vi "GyroSampleSensorLoop.vi"   [LabVIEW 2018]
uses:
  GyroRxLoopData.ctl
  GyroRxLoopStates.ctl
  GyroSBITSample.ctl
  GyroLBITSample.ctl
  GyroSample.ctl
  GyroErrorSample.ctl
  GyroErrorCodes.ctl
  <vilib>/Platform/TimedLoop/XDataNode/timing_clust.ctl
  <vilib>/Platform/TimedLoop/XDataNode/nitl_modes.ctl
  <vilib>/Platform/TimedLoop/XDataNode/wakeup.ctl
  <vilib>/rvi/Emulation/niFpgaSctlEmulationGetInTimedLoop.vi
  <vilib>/rvi/Emulation/niFpgaEmulationReportErrorSimple.vi
  <vilib>/rvi/Emulation/niFpgaGetClockAttributes.vi
  <vilib>/rvi/Emulation/niFpgaCriticalErrorInLSC.vi
  <vilib>/rvi/Emulation/niFpgaEmulationIsFPGAContextNoSignature.vi
  <vilib>/rvi/errors/niFpgaSetErrorForExecOnDevCompSimple.vi
  <vilib>/rvi/eio/common/nirviEmuReportErrorAndStop.vi
  <vilib>/rvi/DataTransferAndStorage/Container/Common/niFpgaContainerGetUniqueNameForEmu.vi
  <vilib>/rvi/FIFO/Fifo_Resource/nirvififoEmulationSetSize.vi
  <vilib>/rvi/FIFO/Fifo_Resource/nirviFifoEmulationQueueMgr.vi
  <instcachedir>/0/nirviFifoEmulationQueueMgr_E5CAEC123FF24DC58D834DCA3CDAA9B5.lvgen/nirviFifoEmulationQueueMgr_E5CAEC123FF24DC58D834DCA3CDAA9B5_001.vi
  <vilib>/Utility/error.llb/Clear Errors.vi
  <vilib>/rvi/FIFO/Fifo_Resource/nirvififoEmulationCreateLock.vi
  <vilib>/rvi/Emulation/niFpgaProcessEmulError.vi
  <vilib>/rvi/FIFO/Fifo_Resource/nirvififoEmulationObtainLock.vi
  <vilib>/rvi/FIFO/Fifo_Resource/nirvififoEmulationReleaseLock.vi
  <vilib>/rvi/occurrence/nirviWaitOnOccurrenceBase.vi
  <vilib>/rvi/errors/nirviReportUnexpectedCaseInternalError.vi
  <vilib>/rvi/errors/nirviReportUnexpectedCaseInternalError (U32).vi
  <vilib>/rvi/eio/common/nirviEmuTemplateMethod_errors.vi
  <vilib>/rvi/Memory/Memory_Emulation/niFpgaMemoryEmulationCacheClearOnFirstRun.vi
  <vilib>/rvi/Memory/Memory_Emulation/nirvimemoryEmulationManagerCache_MakeExclusive.vi
  <vilib>/rvi/Memory/Memory_Emulation/niFpgaMemoryEmulationValidateCache.vi
  <vilib>/rvi/Memory/Memory_Emulation/nirvimemoryEmulationManagerCache_InsertValue.vi
  <vilib>/rvi/Memory/Memory_Emulation/nirvimemoryEmulationManagerCache_ReleaseExclusive.vi
  <vilib>/rvi/Memory/Memory_Emulation/nirvimemoryEmulationManagerCache_GetValue.vi
  <vilib>/rvi/Memory/Memory_Emulation/nirvimemoryEmulationManagerCache_SetValue.vi
  <vilib>/rvi/FIFO/Fifo_Resource/nirvififoEmulationDetermineInputValidOut.vi
  <instcachedir>/0/nirviFifoEmulationQueueMgr_E5CAEC123FF24DC58D834DCA3CDAA9B5.lvgen/nirviFifoEmulationQueueMgr_E5CAEC123FF24DC58D834DCA3CDAA9B5_009.vi
  <instcachedir>/0/nirviFifoEmulationQueueMgr_E5CAEC123FF24DC58D834DCA3CDAA9B5.lvgen/nirviFifoEmulationQueueMgr_E5CAEC123FF24DC58D834DCA3CDAA9B5_010.vi
  <instcachedir>/0/nirviFifoEmulationQueueMgr_E5CAEC123FF24DC58D834DCA3CDAA9B5.lvgen/nirviFifoEmulationQueueMgr_E5CAEC123FF24DC58D834DCA3CDAA9B5_002.vi
  <instcachedir>/0/nirviFifoEmulationQueueMgr_E5CAEC123FF24DC58D834DCA3CDAA9B5.lvgen/nirviFifoEmulationQueueMgr_E5CAEC123FF24DC58D834DCA3CDAA9B5_008.vi
  <instcachedir>/0/nirviFifoEmulationQueueMgr_E5CAEC123FF24DC58D834DCA3CDAA9B5.lvgen/nirviFifoEmulationQueueMgr_E5CAEC123FF24DC58D834DCA3CDAA9B5_011.vi
  <instcachedir>/0/nirviFifoEmulationQueueMgr_E5CAEC123FF24DC58D834DCA3CDAA9B5.lvgen/nirviFifoEmulationQueueMgr_E5CAEC123FF24DC58D834DCA3CDAA9B5_012.vi
  <vilib>/Platform/TimedLoop/XDataNode/XDataNode.xnode
  <vilib>/rvi/DataTransferAndStorage/Container/XNode/niFpgaContainer.xnode
  <vilib>/rvi/FIFO/Fifo_Resource/nirvififoEmulationRead.vi
  <vilib>/eio/EIONode/EIONode.xnode
  <vilib>/rvi/DataTransferAndStorage/Register/Emulation/niFpgaRegisterEmulation.vi
  <vilib>/rvi/FIFO/Fifo_Resource/nirvififoEmulationWrite.vi
  <vilib>/Platform/TimedLoop/XDataNode/XDNodeRunTimeDep.lvlib
types:
  T1 = typedef "GyroRxLoopData.ctl" = cluster{"State":T2, "Timestamp":u64, "Timeout":i32, "CRC":u32, "Checksum":u8, "IsLBIT":bool, "ReservedCount":u8, "SBITSample":T3, "LBITSample":T4, "Sample":T5, "ErrorSample":T6}
  T2 = typedef "GyroRxLoopStates.ctl" = enum16{"WaitForSilence", "ReadHeader3", "IgnoreASCIIResponse", "ReadNormalHeader2", "ReadNormalHeader1", "ReadBITHeader0", "ReadBIT0", "ReadBIT1", "ReadBIT2", "ReadBIT3", "ReadBIT4", "ReadBIT5", "ReadBIT6", "ReadBIT7", "ReadChecksum", "PrepareSBIT", "MoveSBIT", "PrepareLBIT", "MoveLBIT", "ReadSampleHeader0", "ReadSampleX3", "ReadSampleX2", "ReadSampleX1", "ReadSampleX0", "ReadSampleY3", "ReadSampleY2", "ReadSampleY1", "ReadSampleY0", "ReadSampleZ3", "ReadSampleZ2", "ReadSampleZ1", "ReadSampleZ0", "ReadSampleReserved", "ReadSampleStatus", "ReadSampleSequenceNumber", "ReadSampleTemperature1", "ReadSampleTemperature0", "ReadSampleCRC3", "ReadSampleCRC2", "ReadSampleCRC1", "ReadSampleCRC0", "VerifyCRC", "PrepareSample", "MoveSample", "ResponseHeaderError", "ResponseCRCError", "ResponseTimeoutError", "ResponseChecksumError", "PrepareErrorCode", "MoveErrorCode", "ClearCRC", "WaitForCRCCleared"}
  T3 = typedef "GyroSBITSample.ctl" = cluster{"Timestamp":u64, "TxBytes":u64, "RxBytes":u64, "TxFrames":u64, "RxFrames":u64, "BIT0":u8, "BIT1":u8, "BIT2":u8, "BIT3":u8, "BIT4":u8, "BIT5":u8}
  T4 = typedef "GyroLBITSample.ctl" = cluster{"Timestamp":u64, "TxBytes":u64, "RxBytes":u64, "TxFrames":u64, "RxFrames":u64, "BIT0":u8, "BIT1":u8, "BIT2":u8, "BIT3":u8, "BIT4":u8, "BIT5":u8, "BIT6":u8, "BIT7":u8}
  T5 = typedef "GyroSample.ctl" = cluster{"Timestamp":u64, "TxBytes":u64, "RxBytes":u64, "TxFrames":u64, "RxFrames":u64, "GyroX":u32, "GyroY":u32, "GyroZ":u32, "Status":u8, "SequenceNumber":u8, "Temperature":i16}
  T6 = typedef "GyroErrorSample.ctl" = cluster{"Timestamp":u64, "TxBytes":u64, "RxBytes":u64, "TxFrames":u64, "RxFrames":u64, "ErrorCode":T7}
  T7 = typedef "GyroErrorCodes.ctl" = enum8{"None", "ResponseHeaderError", "ResponseCRCError", "ResponseTimeoutError", "ResponseChecksumError"}
  T8 = typedef "XDNodeRunTimeDep.lvlib/timing_clust.ctl" = cluster{"Expected End [f-1]":u64, "Actual End [f-1]":u64, "Finished Late? [f-1]":bool, "Expected End [i-1]":u64, "Actual End [i-1]":u64, "Finished Late? [i-1]":bool, "Expected Start [i]":u64, "Actual Start [i]":u64, "Expected Start [f]":u64, "Actual Start [f]":u64, "Source Name":string, "Structure Name":string, "Period":i64, "Deadline":i64, "Offset":i64, "Start":i64, "Priority":i32, "Timeout":i32, "Mode":T9, "Wakeup Reason":T10, "Error":errorcluster, "Source Type":string, "Secondary Source Type":string, "Global End Time":u64, "Global Start Time":u64, "Frame Duration":u64, "Iteration Duration":u64, "Assigned CPU":i32, "I/O Scan Engine Mode":u32}
  T9 = typedef "XDNodeRunTimeDep.lvlib/nitl_modes.ctl" = enum32{"No Change", "Process missed periods, maintain original phase", "Discard missed periods, maintain original phase", "Process missed periods, ignore original phase", "Discard missed periods, ignore original phase"}
  T10 = typedef "XDNodeRunTimeDep.lvlib/wakeup.ctl" = enum32{"Normal", "Aborted", "Asynchronous wakeup", "Timing source error", "Timed loop error", "Timeout"}
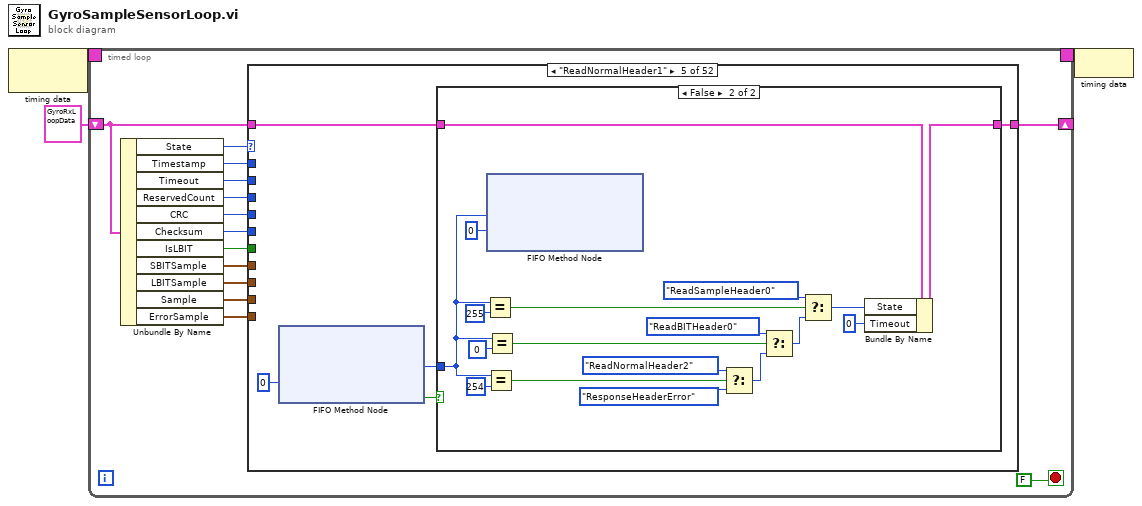
[diagram p0: block diagram]
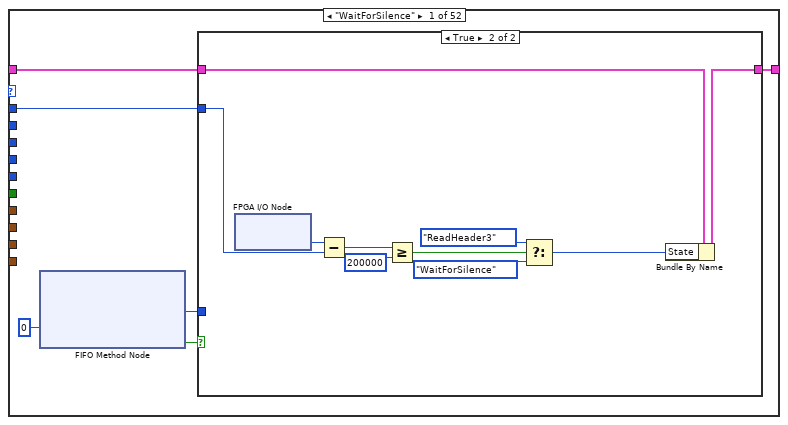
[diagram p2: hidden frame]
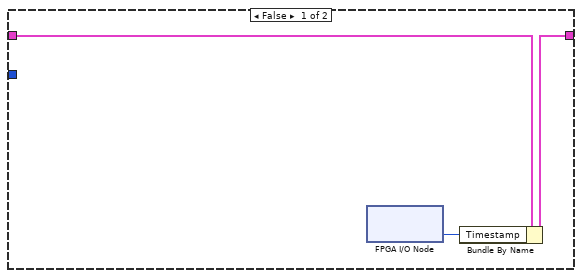
[diagram p3: hidden frame]
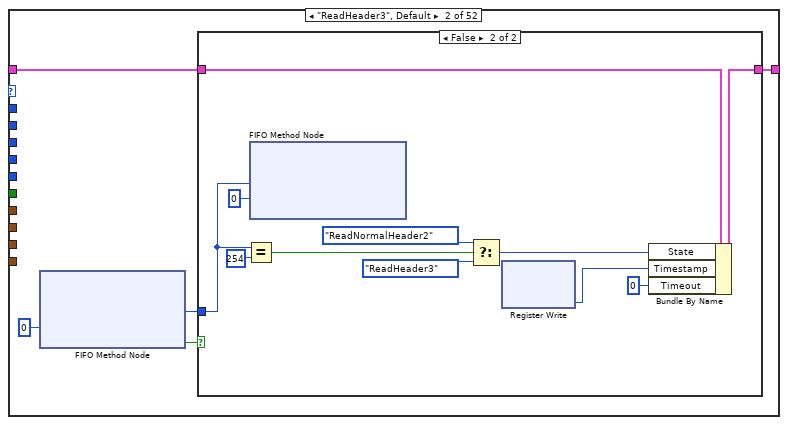
[diagram p4: hidden frame]
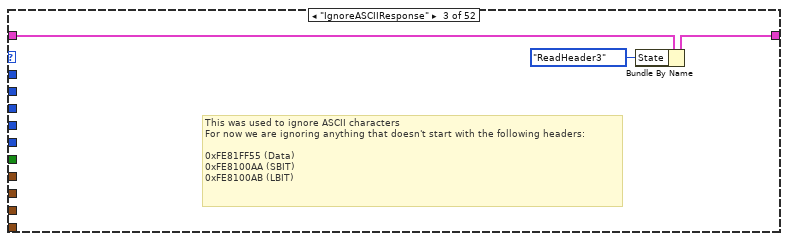
[diagram p6: hidden frame]
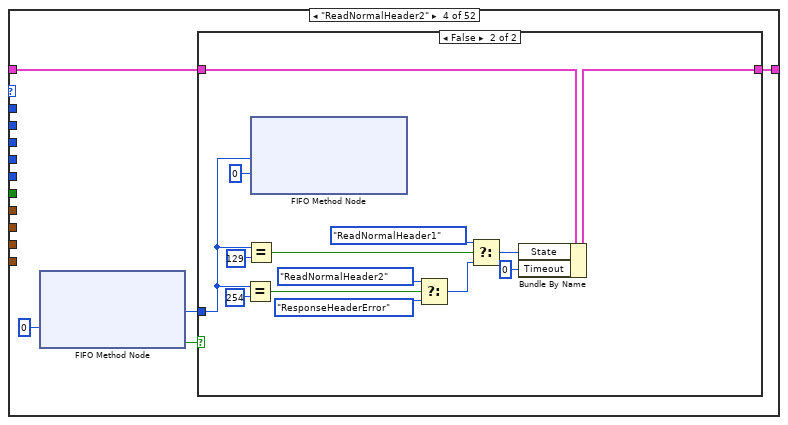
[diagram p7: hidden frame]
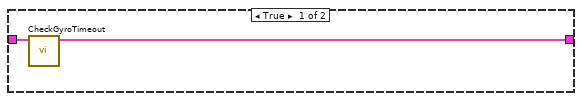
[diagram p8: hidden frame]
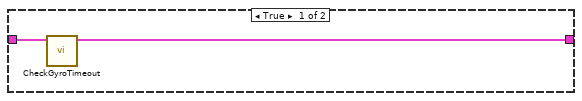
[diagram p9: hidden frame]
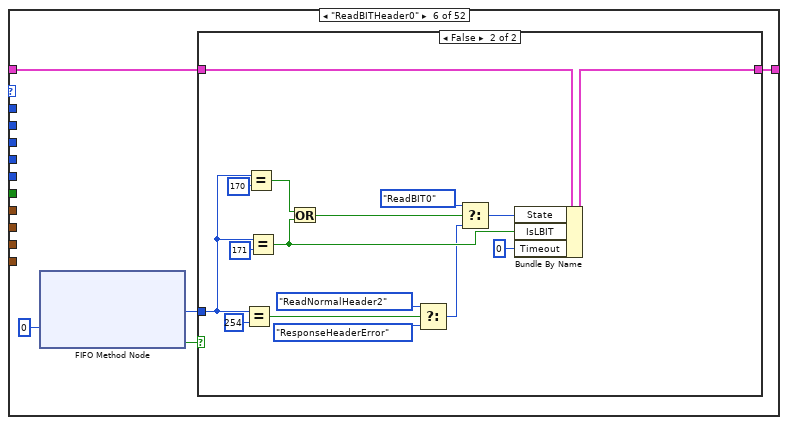
[diagram p10: hidden frame]
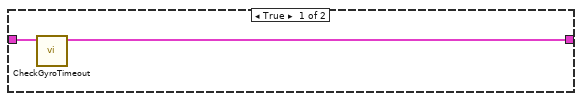
[diagram p11: hidden frame]
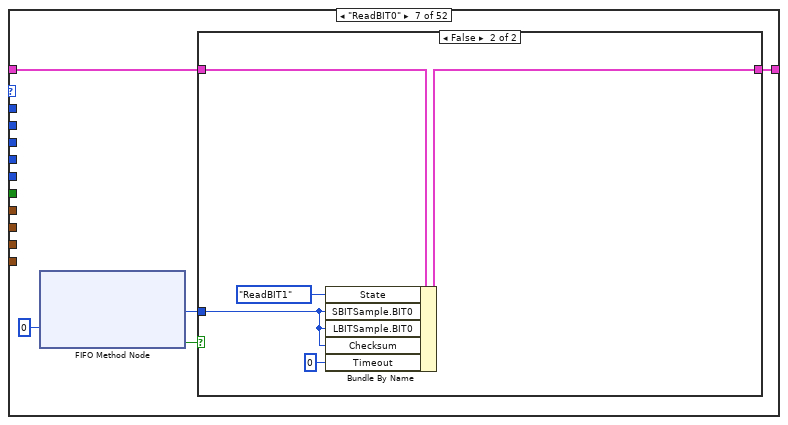
[diagram p12: hidden frame]
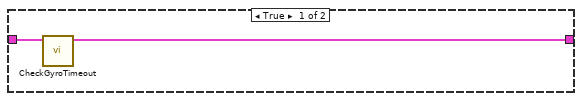
[diagram p13: hidden frame]
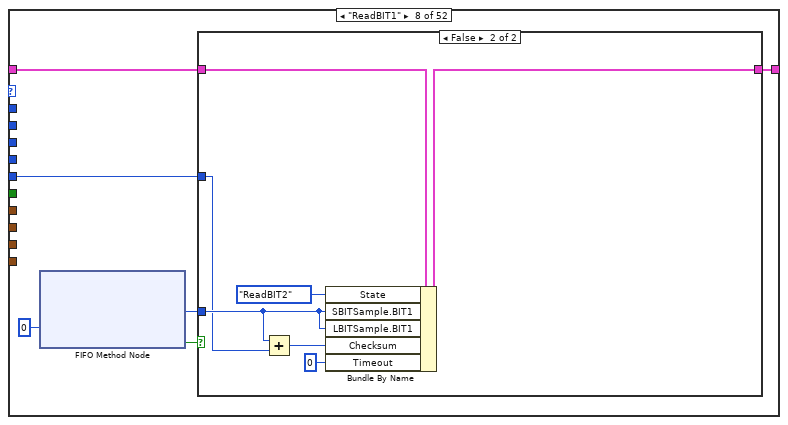
[diagram p14: hidden frame]
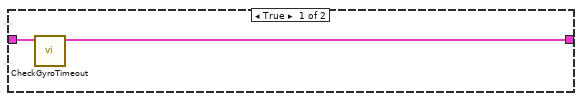
[diagram p15: hidden frame]
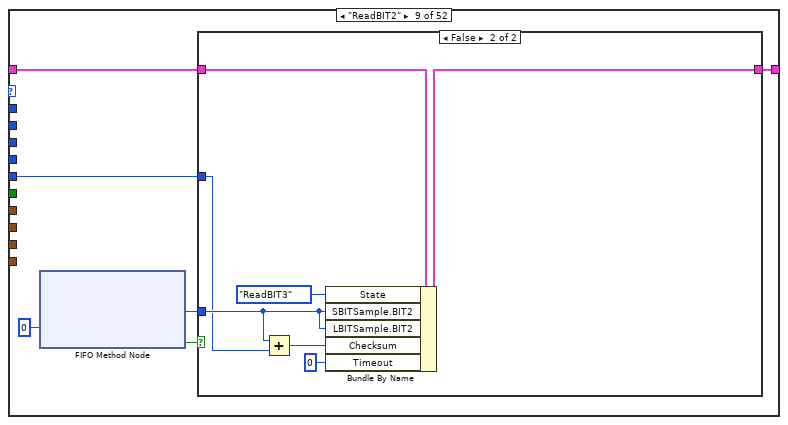
[diagram p16: hidden frame]
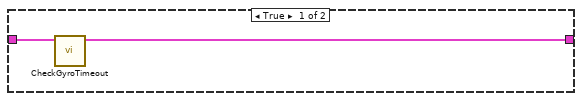
[diagram p17: hidden frame]
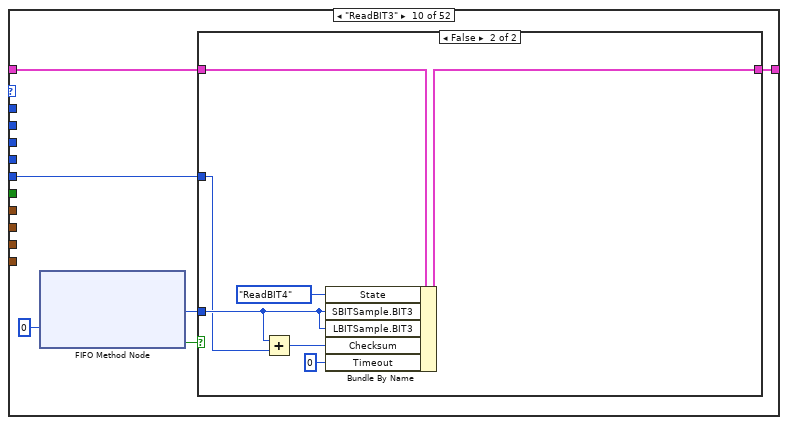
[diagram p18: hidden frame]
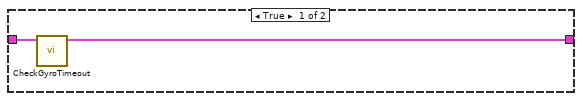
[diagram p19: hidden frame]
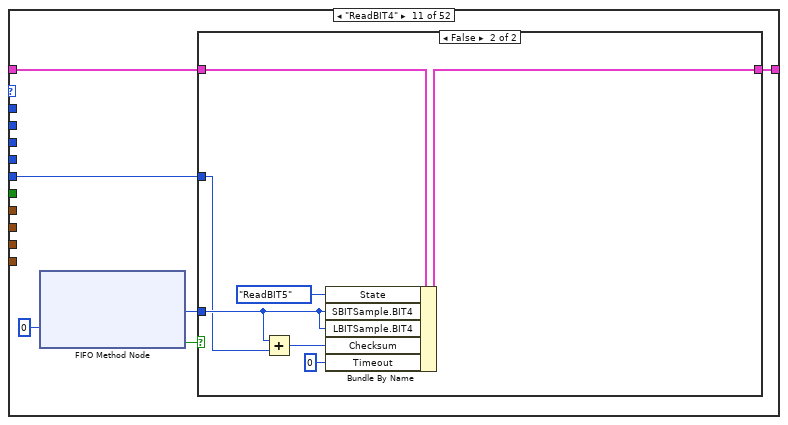
[diagram p20: hidden frame]
diagram:
  n1 = node-c288() -> (w3:T8)  [unwired: 1 in]
  n2 = timed-loop {
    timing: w3 -> [_]
    timing-out: [_] -> w2
    shift-right: [w17] -> _
    shift-left: T1 {"State"=enum."WaitForSilence", "Timestamp"=0, "Timeout"=0, "CRC"=0, "Checksum"=0, "IsLBIT"=FALSE, "ReservedCount"=0, "SBITSample"={"Timestamp"=0, "TxBytes"=0, "RxBytes"=0, "TxFrames"=0, "RxFrames"=0, "BIT0"=0, "BIT1"=0, "BIT2"=0, "BIT3"=0, "BIT4"=0, "BIT5"=0}, "LBITSample"={"Timestamp"=0, "TxBytes"=0, "RxBytes"=0, "TxFrames"=0, "RxFrames"=0, "BIT0"=0, "BIT1"=0, "BIT2"=0, "BIT3"=0, "BIT4"=0, "BIT5"=0, "BIT6"=0, "BIT7"=0}, "Sample"={"Timestamp"=0, "TxBytes"=0, "RxBytes"=0, "TxFrames"=0, "RxFrames"=0, "GyroX"=0, "GyroY"=0, "GyroZ"=0, "Status"=0, "SequenceNumber"=0, "Temperature"=0}, "ErrorSample"={"Timestamp"=0, "TxBytes"=0, "RxBytes"=0, "TxFrames"=0, "RxFrames"=0, "ErrorCode"=enum."None"}} ("GyroRxLoopData") -> [w16]
    stop <- FALSE stop-if-true
    n3 = Unbundle By Name(w16) -> ("State"=w15:T2, "Timestamp"=w14:u64, "Timeout"=w13:i32, "ReservedCount"=w9:u8, "CRC"=w12:u32, "Checksum"=w11:u8, "IsLBIT"=w10:bool, "SBITSample"=w8:T3, "LBITSample"=w7:T4, "Sample"=w6:T5, "ErrorSample"=w5:T6)
    n4 = case shown="\"ReadNormalHeader1\"" w15 {
      tunnel: [w19 w37 w55 w57 w78 w103 w126 w139 w154 w169 w184 w200 w218 w233 w249 w276 w281 w289 w294 w296 w317 w333 w351 w369 w385 w401 w419 w437 w453 w469 w487 w505 w523 w542 w555 w568 w584 w600 w618 w636 w654 w670 w692 w697 w701 w705 w709 w713 w721 w726 w731 w738] -> w17
      tunnel: w16 -> [w20 w38 w56 w58 w79 w104 w127 w140 w155 w170 w185 w201 w219 w234 w250 w277 w282 w290 w295 w297 w318 w334 w352 w370 w386 w402 w420 w438 w454 w470 w488 w506 w524 w543 w556 w569 w585 w601 w619 w637 w655 w671 w693 w698 w702 w706 w710 w714 w722 w727 w732 w739]
      tunnel: w14 -> [w18 _ _ _ _ _ _ _ _ _ _ _ _ _ _ w274 _ w287 _ _ _ _ _ _ _ _ _ _ _ _ _ _ _ _ _ _ _ _ _ _ _ _ w690 _ _ _ _ _ w719 _ _ _]
      tunnel: w13 -> [_ _ _ _ _ _ _ _ _ _ _ _ _ _ _ _ _ _ _ _ _ _ _ _ _ _ _ _ _ _ _ _ _ _ _ _ _ _ _ _ _ _ _ _ _ _ _ _ _ _ _ _]
      tunnel: w12 -> [_ _ _ _ _ _ _ _ _ _ _ _ _ _ _ _ _ _ _ _ _ _ _ _ _ _ _ _ _ _ _ _ _ _ _ _ _ _ w617 w635 w653 w669 _ _ _ _ _ _ _ _ _ _]
      tunnel: w11 -> [_ _ _ _ _ _ _ w138 w153 w168 w183 w199 w217 w232 w248 _ _ _ _ _ _ _ _ _ _ _ _ _ _ _ _ _ _ _ _ _ _ _ _ _ _ _ _ _ _ _ _ _ _ _ _ _]
      tunnel: w10 -> [_ _ _ _ _ _ _ _ _ _ _ w198 _ _ w247 _ _ _ _ _ _ _ _ _ _ _ _ _ _ _ _ _ _ _ _ _ _ _ _ _ _ _ _ _ _ _ _ _ _ _ _ _]
      tunnel: w9 -> [_ _ _ _ _ _ _ _ _ _ _ _ _ _ _ _ _ _ _ _ _ _ _ _ _ _ _ _ _ _ _ _ w522 _ _ _ _ _ _ _ _ _ _ _ _ _ _ _ _ _ _ _]
      tunnel: w8 -> [_ _ _ _ _ _ _ _ _ _ _ _ _ _ _ _ w278 _ _ _ _ _ _ _ _ _ _ _ _ _ _ _ _ _ _ _ _ _ _ _ _ _ _ _ _ _ _ _ _ _ _ _]
      tunnel: w7 -> [_ _ _ _ _ _ _ _ _ _ _ _ _ _ _ _ _ _ w291 _ _ _ _ _ _ _ _ _ _ _ _ _ _ _ _ _ _ _ _ _ _ _ _ _ _ _ _ _ _ _ _ _]
      tunnel: w6 -> [_ _ _ _ _ _ _ _ _ _ _ _ _ _ _ _ _ _ _ _ _ _ _ _ _ _ _ _ _ _ _ _ _ _ _ _ _ _ _ _ _ _ _ w695 _ _ _ _ _ _ _ _]
      tunnel: w5 -> [_ _ _ _ _ _ _ _ _ _ _ _ _ _ _ _ _ _ _ _ _ _ _ _ _ _ _ _ _ _ _ _ _ _ _ _ _ _ _ _ _ _ _ _ _ _ _ _ _ w724 _ _]
      frame "WaitForSilence" {
        n5 = xnode ("FIFO Method Node")("Timeout"=0) -> ("Element"=w22:u8, "Timed Out?"=w21:bool)  [unwired: 1 in, 1 out]
        n6 = case shown="True" w21 {
          tunnel: w22 -> [_ _]
          tunnel: w20 -> [w26 w36]
          tunnel: [w25 w35] -> w19
          tunnel: w18 -> [_ w33]
          frame False {
            n7 = xnode "FPGA I/O Node"() -> ("Time"=w24:u64)  [unwired: 1 in, 1 out]
            n8 = Bundle By Name(cluster=w26, "Timestamp"=w24) -> (w25:T1)
          }
          frame True {
            n9 = xnode "FPGA I/O Node"() -> ("Time"=w34:u64)  [unwired: 1 in, 1 out]
            n10 = Subtract(x=w34, y=w33) -> (x-y=w32:u64)
            n11 = Greater Or Equal?(x=w32, y=u64 200000) -> (x >= y?=w30:bool)
            n12 = Select(t=GyroRxLoopStates."ReadHeader3" ("State"), s=w30, f=GyroRxLoopStates."WaitForSilence" ("State")) -> (s? t:f=w27:T2)
            n13 = Bundle By Name(cluster=w36, "State"=w27) -> (w35:T1)
          }
        }
      }
      frame "ReadHeader3", Default {
        n14 = xnode ("FIFO Method Node")("Timeout"=0) -> ("Element"=w40:u8, "Timed Out?"=w39:bool)  [unwired: 1 in, 1 out]
        n15 = case shown="False" w39 {
          tunnel: w40 -> [_ w47]
          tunnel: w38 -> [w42 w50]
          tunnel: [w42 w49] -> w37
          frame True {
          }
          frame False {
            n16 = Equal?(x=w47, y=u8 254) -> (x = y?=w51:bool)
            n17 = xnode ("FIFO Method Node")("Element"=w47, "Timeout"=0) -> ()  [unwired: 1 in, 2 out]
            n18 = Select(t=GyroRxLoopStates."ReadNormalHeader2", s=w51, f=GyroRxLoopStates."ReadHeader3" ("t")) -> (s? t:f=w48:T2)
            n19 = xnode "Register Write"() -> ("Data"=w43:u64)  [unwired: 1 in, 1 out]
            n20 = Bundle By Name(cluster=w50, "State"=w48, "Timestamp"=w43, "Timeout"=0) -> (w49:T1)
          }
        }
      }
      frame "IgnoreASCIIResponse" {
        # "This was used to ignore ASCII characters\nFor now we are ignoring anything that doesn't start with the following headers:\n\n0xFE81FF55 (Data)\n0xFE8100AA (SBIT)\n0xFE8100AB (LBIT)"
        n21 = Bundle By Name(cluster=w56, "State"=GyroRxLoopStates."ReadHeader3") -> (w55:T1)
      }
      frame "ReadNormalHeader2" {
        n22 = xnode ("FIFO Method Node")("Timeout"=0) -> ("Element"=w60:u8, "Timed Out?"=w59:bool)  [unwired: 1 in, 1 out]
        n23 = case shown="False" w59 {
          tunnel: w60 -> [_ w69]
          tunnel: w58 -> [w63 w74]
          tunnel: [w62 w73] -> w57
          frame True {
            n24 = call "CheckGyroTimeout.vi"("GyroRxLoopData in"=w63) -> ("GyroRxLoopData out"=w62:T1)  [unwired: 10 in]
          }
          frame False {
            n25 = Equal?(x=w69, y=u8 254) -> (x = y?=w67:bool)
            n26 = Equal?(x=w69, y=u8 129) -> (x = y?=w75:bool)
            n27 = xnode ("FIFO Method Node")("Element"=w69, "Timeout"=0) -> ()  [unwired: 1 in, 2 out]
            n28 = Select(t=GyroRxLoopStates."ReadNormalHeader2", s=w67, f=GyroRxLoopStates."ResponseHeaderError") -> (s? t:f=w66:T2)
            n29 = Select(t=GyroRxLoopStates."ReadNormalHeader1", s=w75, f=w66) -> (s? t:f=w72:T2)
            n30 = Bundle By Name(cluster=w74, "State"=w72, "Timeout"=0) -> (w73:T1)
          }
        }
      }
      frame "ReadNormalHeader1" {
        n31 = xnode ("FIFO Method Node")("Timeout"=0) -> ("Element"=w81:u8, "Timed Out?"=w80:bool)  [unwired: 1 in, 1 out]
        n32 = case shown="False" w80 {
          tunnel: w81 -> [_ w87]
          tunnel: w79 -> [w84 w99]
          tunnel: [w83 w98] -> w78
          frame True {
            n33 = call "CheckGyroTimeout.vi"("GyroRxLoopData in"=w84) -> ("GyroRxLoopData out"=w83:T1)  [unwired: 10 in]
          }
          frame False {
            n34 = Equal?(x=w87, y=u8 255) -> (x = y?=w100:bool)
            n35 = Equal?(x=w87, y=u8 254) -> (x = y?=w90:bool)
            n36 = xnode ("FIFO Method Node")("Element"=w87, "Timeout"=0) -> ()  [unwired: 1 in, 2 out]
            n37 = Equal?(x=w87, y=u8 0) -> (x = y?=w95:bool)
            n38 = Select(t=GyroRxLoopStates."ReadNormalHeader2", s=w90, f=GyroRxLoopStates."ResponseHeaderError") -> (s? t:f=w86:T2)
            n39 = Select(t=GyroRxLoopStates."ReadBITHeader0" ("f"), s=w95, f=w86) -> (s? t:f=w93:T2)
            n40 = Select(t=GyroRxLoopStates."ReadSampleHeader0", s=w100, f=w93) -> (s? t:f=w97:T2)
            n41 = Bundle By Name(cluster=w99, "State"=w97, "Timeout"=0) -> (w98:T1)
          }
        }
      }
      frame "ReadBITHeader0" {
        n42 = xnode ("FIFO Method Node")("Timeout"=0) -> ("Element"=w106:u8, "Timed Out?"=w105:bool)  [unwired: 1 in, 1 out]
        n43 = case shown="False" w105 {
          tunnel: w106 -> [_ w113]
          tunnel: w104 -> [w109 w123]
          tunnel: [w108 w122] -> w103
          frame True {
            n44 = call "CheckGyroTimeout.vi"("GyroRxLoopData in"=w109) -> ("GyroRxLoopData out"=w108:T1)  [unwired: 10 in]
          }
          frame False {
            n45 = Equal?(x=w113, y=u8 254) -> (x = y?=w115:bool)
            n46 = Equal?(x=w113, y=u8 170) -> (x = y?=w119:bool)
            n47 = Equal?(x=w113, y=u8 171) -> (x = y?=w117:bool)
            n48 = Or(x=w119, y=w117) -> (x .or. y?=w118:bool)
            n49 = Select(t=GyroRxLoopStates."ReadNormalHeader2", s=w115, f=GyroRxLoopStates."ResponseHeaderError") -> (s? t:f=w111:T2)
            n50 = Select(t=GyroRxLoopStates."ReadBIT0", s=w118, f=w111) -> (s? t:f=w121:T2)
            n51 = Bundle By Name(cluster=w123, "State"=w121, "IsLBIT"=w117, "Timeout"=0) -> (w122:T1)
          }
        }
      }
      frame "ReadBIT0" {
        n52 = xnode ("FIFO Method Node")("Timeout"=0) -> ("Element"=w129:u8, "Timed Out?"=w128:bool)  [unwired: 1 in, 1 out]
        n53 = case shown="False" w128 {
          tunnel: w129 -> [_ w134]
          tunnel: w127 -> [w132 w137]
          tunnel: [w131 w136] -> w126
          frame True {
            n54 = call "CheckGyroTimeout.vi"("GyroRxLoopData in"=w132) -> ("GyroRxLoopData out"=w131:T1)  [unwired: 10 in]
          }
          frame False {
            n55 = Bundle By Name(cluster=w137, "State"=GyroRxLoopStates."ReadBIT1" ("t"), "SBITSample.BIT0"=w134, "LBITSample.BIT0"=w134, "Checksum"=w134, "Timeout"=0) -> (w136:T1)
          }
        }
      }
      frame "ReadBIT1" {
        n56 = xnode ("FIFO Method Node")("Timeout"=0) -> ("Element"=w142:u8, "Timed Out?"=w141:bool)  [unwired: 1 in, 1 out]
        n57 = case shown="False" w141 {
          tunnel: w142 -> [_ w149]
          tunnel: w140 -> [w145 w152]
          tunnel: [w144 w151] -> w139
          tunnel: w138 -> [_ w148]
          frame True {
            n58 = call "CheckGyroTimeout.vi"("GyroRxLoopData in"=w145) -> ("GyroRxLoopData out"=w144:T1)  [unwired: 10 in]
          }
          frame False {
            n59 = Add(x=w149, y=w148) -> (x+y=w147:u8)
            n60 = Bundle By Name(cluster=w152, "State"=GyroRxLoopStates."ReadBIT2" ("t"), "SBITSample.BIT1"=w149, "LBITSample.BIT1"=w149, "Checksum"=w147, "Timeout"=0) -> (w151:T1)
          }
        }
      }
      frame "ReadBIT2" {
        n61 = xnode ("FIFO Method Node")("Timeout"=0) -> ("Element"=w157:u8, "Timed Out?"=w156:bool)  [unwired: 1 in, 1 out]
        n62 = case shown="False" w156 {
          tunnel: w157 -> [_ w164]
          tunnel: w155 -> [w160 w167]
          tunnel: [w159 w166] -> w154
          tunnel: w153 -> [_ w163]
          frame True {
            n63 = call "CheckGyroTimeout.vi"("GyroRxLoopData in"=w160) -> ("GyroRxLoopData out"=w159:T1)  [unwired: 10 in]
          }
          frame False {
            n64 = Add(x=w164, y=w163) -> (x+y=w162:u8)
            n65 = Bundle By Name(cluster=w167, "State"=GyroRxLoopStates."ReadBIT3" ("t"), "SBITSample.BIT2"=w164, "LBITSample.BIT2"=w164, "Checksum"=w162, "Timeout"=0) -> (w166:T1)
          }
        }
      }
      frame "ReadBIT3" {
        n66 = xnode ("FIFO Method Node")("Timeout"=0) -> ("Element"=w172:u8, "Timed Out?"=w171:bool)  [unwired: 1 in, 1 out]
        n67 = case shown="False" w171 {
          tunnel: w172 -> [_ w179]
          tunnel: w170 -> [w175 w182]
          tunnel: [w174 w181] -> w169
          tunnel: w168 -> [_ w178]
          frame True {
            n68 = call "CheckGyroTimeout.vi"("GyroRxLoopData in"=w175) -> ("GyroRxLoopData out"=w174:T1)  [unwired: 10 in]
          }
          frame False {
            n69 = Add(x=w179, y=w178) -> (x+y=w177:u8)
            n70 = Bundle By Name(cluster=w182, "State"=GyroRxLoopStates."ReadBIT4" ("t"), "SBITSample.BIT3"=w179, "LBITSample.BIT3"=w179, "Checksum"=w177, "Timeout"=0) -> (w181:T1)
          }
        }
      }
      frame "ReadBIT4" {
        n71 = xnode ("FIFO Method Node")("Timeout"=0) -> ("Element"=w187:u8, "Timed Out?"=w186:bool)  [unwired: 1 in, 1 out]
        n72 = case shown="False" w186 {
          tunnel: w187 -> [_ w194]
          tunnel: w185 -> [w190 w197]
          tunnel: [w189 w196] -> w184
          tunnel: w183 -> [_ w193]
          frame True {
            n73 = call "CheckGyroTimeout.vi"("GyroRxLoopData in"=w190) -> ("GyroRxLoopData out"=w189:T1)  [unwired: 10 in]
          }
          frame False {
            n74 = Add(x=w194, y=w193) -> (x+y=w192:u8)
            n75 = Bundle By Name(cluster=w197, "State"=GyroRxLoopStates."ReadBIT5" ("t"), "SBITSample.BIT4"=w194, "LBITSample.BIT4"=w194, "Checksum"=w192, "Timeout"=0) -> (w196:T1)
          }
        }
      }
      frame "ReadBIT5" {
        n76 = xnode ("FIFO Method Node")("Timeout"=0) -> ("Element"=w203:u8, "Timed Out?"=w202:bool)  [unwired: 1 in, 1 out]
        n77 = case shown="False" w202 {
          tunnel: w203 -> [_ w214]
          tunnel: w201 -> [w206 w216]
          tunnel: [w205 w215] -> w200
          tunnel: w199 -> [_ w213]
          tunnel: w198 -> [_ w211]
          frame True {
            n78 = call "CheckGyroTimeout.vi"("GyroRxLoopData in"=w206) -> ("GyroRxLoopData out"=w205:T1)  [unwired: 10 in]
          }
          frame False {
            n79 = Add(x=w214, y=w213) -> (x+y=w212:u8)
            n80 = Select(t=GyroRxLoopStates."ReadBIT6", s=w211, f=GyroRxLoopStates."ReadChecksum") -> (s? t:f=w208:T2)
            n81 = Bundle By Name(cluster=w216, "State"=w208, "SBITSample.BIT5"=w214, "LBITSample.BIT5"=w214, "Checksum"=w212, "Timeout"=0) -> (w215:T1)
          }
        }
      }
      frame "ReadBIT6" {
        n82 = xnode ("FIFO Method Node")("Timeout"=0) -> ("Element"=w221:u8, "Timed Out?"=w220:bool)  [unwired: 1 in, 1 out]
        n83 = case shown="False" w220 {
          tunnel: w221 -> [_ w229]
          tunnel: w219 -> [w224 w231]
          tunnel: [w223 w230] -> w218
          tunnel: w217 -> [_ w228]
          frame True {
            n84 = call "CheckGyroTimeout.vi"("GyroRxLoopData in"=w224) -> ("GyroRxLoopData out"=w223:T1)  [unwired: 10 in]
          }
          frame False {
            n85 = Add(x=w229, y=w228) -> (x+y=w227:u8)
            n86 = Bundle By Name(cluster=w231, "State"=GyroRxLoopStates."ReadBIT7" ("t"), "LBITSample.BIT6"=w229, "Checksum"=w227, "Timeout"=0) -> (w230:T1)
          }
        }
      }
      frame "ReadBIT7" {
        n87 = xnode ("FIFO Method Node")("Timeout"=0) -> ("Element"=w236:u8, "Timed Out?"=w235:bool)  [unwired: 1 in, 1 out]
        n88 = case shown="False" w235 {
          tunnel: w236 -> [_ w244]
          tunnel: w234 -> [w239 w246]
          tunnel: [w238 w245] -> w233
          tunnel: w232 -> [_ w243]
          frame True {
            n89 = call "CheckGyroTimeout.vi"("GyroRxLoopData in"=w239) -> ("GyroRxLoopData out"=w238:T1)  [unwired: 10 in]
          }
          frame False {
            n90 = Add(x=w244, y=w243) -> (x+y=w242:u8)
            n91 = Bundle By Name(cluster=w246, "State"=GyroRxLoopStates."ReadChecksum" ("t"), "LBITSample.BIT7"=w244, "Checksum"=w242, "Timeout"=0) -> (w245:T1)
          }
        }
      }
      frame "ReadChecksum" {
        n92 = xnode ("FIFO Method Node")("Timeout"=0) -> ("Element"=w252:u8, "Timed Out?"=w251:bool)  [unwired: 1 in, 1 out]
        n93 = case shown="False" w251 {
          tunnel: w252 -> [_ w265]
          tunnel: w250 -> [w255 w267]
          tunnel: [w254 w266] -> w249
          tunnel: w248 -> [_ w264]
          tunnel: w247 -> [_ w263]
          frame True {
            n94 = call "CheckGyroTimeout.vi"("GyroRxLoopData in"=w255) -> ("GyroRxLoopData out"=w254:T1)  [unwired: 10 in]
          }
          frame False {
            n95 = Not Equal?(x=w264, y=w265) -> (x != y?=w257:bool)
            n96 = Select(t=GyroRxLoopStates."PrepareLBIT", s=w263, f=GyroRxLoopStates."PrepareSBIT" ("t")) -> (s? t:f=w259:T2)
            n97 = case shown="False" w257 {
              frame True {
              }
              frame False {
                n98 = xnode ("Register Read")() -> ("Data"=w269:u64)  [unwired: 1 in, 1 out]
                n99 = Increment(x=w269) -> (x+1=w268:u64)
                n100 = xnode ("Register Write")("Data"=w268) -> ()  [unwired: 1 in, 1 out]
              }
            }
            n101 = Select(t=GyroRxLoopStates."ResponseChecksumError", s=w257, f=w259) -> (s? t:f=w258:T2)
            n102 = Bundle By Name(cluster=w267, "State"=w258, "Timeout"=0) -> (w266:T1)
          }
        }
      }
      frame "PrepareSBIT" {
        n103 = xnode ("Register Read")() -> ("Data"=w273:u64)  [unwired: 1 in, 1 out]
        n104 = xnode ("Register Read")() -> ("Data"=w272:u64)  [unwired: 1 in, 1 out]
        n105 = xnode ("Register Read")() -> ("Data"=w271:u64)  [unwired: 1 in, 1 out]
        n106 = xnode ("Register Read")() -> ("Data"=w270:u64)  [unwired: 1 in, 1 out]
        n107 = Bundle By Name(cluster=w277, "State"=GyroRxLoopStates."MoveSBIT", "SBITSample.Timestamp"=w274, "SBITSample.TxBytes"=w273, "SBITSample.RxBytes"=w272, "SBITSample.TxFrames"=w271, "SBITSample.RxFrames"=w270) -> (w276:T1)
      }
      frame "MoveSBIT" {
        n108 = xnode ("FIFO Method Node")("Element"=w278, "Timeout"=0) -> ()  [unwired: 1 in, 2 out]
        n109 = Bundle By Name(cluster=w282, "State"=GyroRxLoopStates."ClearCRC") -> (w281:T1)
      }
      frame "PrepareLBIT" {
        n110 = xnode ("Register Read")() -> ("Data"=w286:u64)  [unwired: 1 in, 1 out]
        n111 = xnode ("Register Read")() -> ("Data"=w285:u64)  [unwired: 1 in, 1 out]
        n112 = xnode ("Register Read")() -> ("Data"=w284:u64)  [unwired: 1 in, 1 out]
        n113 = xnode ("Register Read")() -> ("Data"=w283:u64)  [unwired: 1 in, 1 out]
        n114 = Bundle By Name(cluster=w290, "State"=GyroRxLoopStates."MoveLBIT", "LBITSample.Timestamp"=w287, "LBITSample.TxBytes"=w286, "LBITSample.RxBytes"=w285, "LBITSample.TxFrames"=w284, "LBITSample.RxFrames"=w283) -> (w289:T1)
      }
      frame "MoveLBIT" {
        n115 = xnode ("FIFO Method Node")("Element"=w291, "Timeout"=0) -> ()  [unwired: 1 in, 2 out]
        n116 = Bundle By Name(cluster=w295, "State"=GyroRxLoopStates."ClearCRC") -> (w294:T1)
      }
      frame "ReadSampleHeader0" {
        n117 = xnode ("FIFO Method Node")("Timeout"=0) -> ("Element"=w299:u8, "Timed Out?"=w298:bool)  [unwired: 1 in, 1 out]
        n118 = case shown="False" w298 {
          tunnel: w299 -> [_ w305]
          tunnel: w297 -> [w302 w314]
          tunnel: [w301 w313] -> w296
          frame True {
            n119 = call "CheckGyroTimeout.vi"("GyroRxLoopData in"=w302) -> ("GyroRxLoopData out"=w301:T1)  [unwired: 10 in]
          }
          frame False {
            n120 = xnode ("FIFO Method Node")("Element"=w305, "Timeout"=0) -> ()  [unwired: 1 in, 2 out]
            n121 = Equal?(x=w305, y=u8 85) -> (x = y?=w311:bool)
            n122 = Equal?(x=w305, y=u8 254) -> (x = y?=w308:bool)
            n123 = Select(t=GyroRxLoopStates."ReadNormalHeader2", s=w308, f=GyroRxLoopStates."ResponseHeaderError") -> (s? t:f=w304:T2)
            n124 = Select(t=GyroRxLoopStates."ReadSampleX3", s=w311, f=w304) -> (s? t:f=w312:T2)
            n125 = Bundle By Name(cluster=w314, "State"=w312, "Timeout"=0) -> (w313:T1)
          }
        }
      }
      frame "ReadSampleX3" {
        n126 = xnode ("FIFO Method Node")("Timeout"=0) -> ("Element"=w320:u8, "Timed Out?"=w319:bool)  [unwired: 1 in, 1 out]
        n127 = case shown="False" w319 {
          tunnel: w320 -> [_ w329]
          tunnel: w318 -> [w323 w326]
          tunnel: [w322 w332] -> w317
          frame True {
            n128 = call "CheckGyroTimeout.vi"("GyroRxLoopData in"=w323) -> ("GyroRxLoopData out"=w322:T1)  [unwired: 10 in]
          }
          frame False {
            n129 = To Unsigned Long Integer(number=w329) -> (unsigned 32bit integer=w328:u32)
            n130 = xnode ("FIFO Method Node")("Element"=w329, "Timeout"=0) -> ()  [unwired: 1 in, 2 out]
            n131 = Logical Shift(y=i16 24, x=w328) -> (x << y=w325:u32)
            n132 = Bundle By Name(cluster=w326, "State"=GyroRxLoopStates."ReadSampleX2" ("t"), "Sample.GyroX"=w325, "Timeout"=0) -> (w332:T1)
          }
        }
      }
      frame "ReadSampleX2" {
        n133 = xnode ("FIFO Method Node")("Timeout"=0) -> ("Element"=w336:u8, "Timed Out?"=w335:bool)  [unwired: 1 in, 1 out]
        n134 = case shown="False" w335 {
          tunnel: w336 -> [_ w347]
          tunnel: w334 -> [w339 w344]
          tunnel: [w338 w350] -> w333
          frame True {
            n135 = call "CheckGyroTimeout.vi"("GyroRxLoopData in"=w339) -> ("GyroRxLoopData out"=w338:T1)  [unwired: 10 in]
          }
          frame False {
            n136 = Unbundle By Name(w344) -> ("Sample.GyroX"=w343:u32)
            n137 = To Unsigned Long Integer(number=w347) -> (unsigned 32bit integer=w346:u32)
            n138 = xnode ("FIFO Method Node")("Element"=w347, "Timeout"=0) -> ()  [unwired: 1 in, 2 out]
            n139 = Logical Shift(y=i16 16, x=w346) -> (x << y=w342:u32)
            n140 = Or(x=w343, y=w342) -> (x .or. y?=w341:u32)
            n141 = Bundle By Name(cluster=w344, "State"=GyroRxLoopStates."ReadSampleX1" ("t"), "Sample.GyroX"=w341, "Timeout"=0) -> (w350:T1)
          }
        }
      }
      frame "ReadSampleX1" {
        n142 = xnode ("FIFO Method Node")("Timeout"=0) -> ("Element"=w354:u8, "Timed Out?"=w353:bool)  [unwired: 1 in, 1 out]
        n143 = case shown="False" w353 {
          tunnel: w354 -> [_ w365]
          tunnel: w352 -> [w357 w362]
          tunnel: [w356 w368] -> w351
          frame True {
            n144 = call "CheckGyroTimeout.vi"("GyroRxLoopData in"=w357) -> ("GyroRxLoopData out"=w356:T1)  [unwired: 10 in]
          }
          frame False {
            n145 = Unbundle By Name(w362) -> ("Sample.GyroX"=w361:u32)
            n146 = To Unsigned Long Integer(number=w365) -> (unsigned 32bit integer=w364:u32)
            n147 = xnode ("FIFO Method Node")("Element"=w365, "Timeout"=0) -> ()  [unwired: 1 in, 2 out]
            n148 = Logical Shift(y=i16 8, x=w364) -> (x << y=w360:u32)
            n149 = Or(x=w361, y=w360) -> (x .or. y?=w359:u32)
            n150 = Bundle By Name(cluster=w362, "State"=GyroRxLoopStates."ReadSampleX0" ("t"), "Sample.GyroX"=w359, "Timeout"=0) -> (w368:T1)
          }
        }
      }
      frame "ReadSampleX0" {
        n151 = xnode ("FIFO Method Node")("Timeout"=0) -> ("Element"=w372:u8, "Timed Out?"=w371:bool)  [unwired: 1 in, 1 out]
        n152 = case shown="False" w371 {
          tunnel: w372 -> [_ w381]
          tunnel: w370 -> [w375 w380]
          tunnel: [w374 w384] -> w369
          frame True {
            n153 = call "CheckGyroTimeout.vi"("GyroRxLoopData in"=w375) -> ("GyroRxLoopData out"=w374:T1)  [unwired: 10 in]
          }
          frame False {
            n154 = Unbundle By Name(w380) -> ("Sample.GyroX"=w379:u32)
            n155 = To Unsigned Long Integer(number=w381) -> (unsigned 32bit integer=w378:u32)
            n156 = xnode ("FIFO Method Node")("Element"=w381, "Timeout"=0) -> ()  [unwired: 1 in, 2 out]
            n157 = Or(x=w379, y=w378) -> (x .or. y?=w377:u32)
            n158 = Bundle By Name(cluster=w380, "State"=GyroRxLoopStates."ReadSampleY3" ("t"), "Sample.GyroX"=w377, "Timeout"=0) -> (w384:T1)
          }
        }
      }
      frame "ReadSampleY3" {
        n159 = xnode ("FIFO Method Node")("Timeout"=0) -> ("Element"=w388:u8, "Timed Out?"=w387:bool)  [unwired: 1 in, 1 out]
        n160 = case shown="False" w387 {
          tunnel: w388 -> [_ w397]
          tunnel: w386 -> [w391 w394]
          tunnel: [w390 w400] -> w385
          frame True {
            n161 = call "CheckGyroTimeout.vi"("GyroRxLoopData in"=w391) -> ("GyroRxLoopData out"=w390:T1)  [unwired: 10 in]
          }
          frame False {
            n162 = To Unsigned Long Integer(number=w397) -> (unsigned 32bit integer=w396:u32)
            n163 = xnode ("FIFO Method Node")("Element"=w397, "Timeout"=0) -> ()  [unwired: 1 in, 2 out]
            n164 = Logical Shift(y=i16 24, x=w396) -> (x << y=w393:u32)
            n165 = Bundle By Name(cluster=w394, "State"=GyroRxLoopStates."ReadSampleY2" ("t"), "Sample.GyroY"=w393, "Timeout"=0) -> (w400:T1)
          }
        }
      }
      frame "ReadSampleY2" {
        n166 = xnode ("FIFO Method Node")("Timeout"=0) -> ("Element"=w404:u8, "Timed Out?"=w403:bool)  [unwired: 1 in, 1 out]
        n167 = case shown="False" w403 {
          tunnel: w404 -> [_ w415]
          tunnel: w402 -> [w407 w412]
          tunnel: [w406 w418] -> w401
          frame True {
            n168 = call "CheckGyroTimeout.vi"("GyroRxLoopData in"=w407) -> ("GyroRxLoopData out"=w406:T1)  [unwired: 10 in]
          }
          frame False {
            n169 = Unbundle By Name(w412) -> ("Sample.GyroY"=w411:u32)
            n170 = To Unsigned Long Integer(number=w415) -> (unsigned 32bit integer=w414:u32)
            n171 = xnode ("FIFO Method Node")("Element"=w415, "Timeout"=0) -> ()  [unwired: 1 in, 2 out]
            n172 = Logical Shift(y=i16 16, x=w414) -> (x << y=w410:u32)
            n173 = Or(x=w411, y=w410) -> (x .or. y?=w409:u32)
            n174 = Bundle By Name(cluster=w412, "State"=GyroRxLoopStates."ReadSampleY1" ("t"), "Sample.GyroY"=w409, "Timeout"=0) -> (w418:T1)
          }
        }
      }
      frame "ReadSampleY1" {
        n175 = xnode ("FIFO Method Node")("Timeout"=0) -> ("Element"=w422:u8, "Timed Out?"=w421:bool)  [unwired: 1 in, 1 out]
        n176 = case shown="False" w421 {
          tunnel: w422 -> [_ w433]
          tunnel: w420 -> [w425 w430]
          tunnel: [w424 w436] -> w419
          frame True {
            n177 = call "CheckGyroTimeout.vi"("GyroRxLoopData in"=w425) -> ("GyroRxLoopData out"=w424:T1)  [unwired: 10 in]
          }
          frame False {
            n178 = Unbundle By Name(w430) -> ("Sample.GyroY"=w429:u32)
            n179 = To Unsigned Long Integer(number=w433) -> (unsigned 32bit integer=w432:u32)
            n180 = xnode ("FIFO Method Node")("Element"=w433, "Timeout"=0) -> ()  [unwired: 1 in, 2 out]
            n181 = Logical Shift(y=i16 8, x=w432) -> (x << y=w428:u32)
            n182 = Or(x=w429, y=w428) -> (x .or. y?=w427:u32)
            n183 = Bundle By Name(cluster=w430, "State"=GyroRxLoopStates."ReadSampleY0" ("t"), "Sample.GyroY"=w427, "Timeout"=0) -> (w436:T1)
          }
        }
      }
      frame "ReadSampleY0" {
        n184 = xnode ("FIFO Method Node")("Timeout"=0) -> ("Element"=w440:u8, "Timed Out?"=w439:bool)  [unwired: 1 in, 1 out]
        n185 = case shown="False" w439 {
          tunnel: w440 -> [_ w449]
          tunnel: w438 -> [w443 w448]
          tunnel: [w442 w452] -> w437
          frame True {
            n186 = call "CheckGyroTimeout.vi"("GyroRxLoopData in"=w443) -> ("GyroRxLoopData out"=w442:T1)  [unwired: 10 in]
          }
          frame False {
            n187 = Unbundle By Name(w448) -> ("Sample.GyroY"=w447:u32)
            n188 = To Unsigned Long Integer(number=w449) -> (unsigned 32bit integer=w446:u32)
            n189 = xnode ("FIFO Method Node")("Element"=w449, "Timeout"=0) -> ()  [unwired: 1 in, 2 out]
            n190 = Or(x=w447, y=w446) -> (x .or. y?=w445:u32)
            n191 = Bundle By Name(cluster=w448, "State"=GyroRxLoopStates."ReadSampleZ3" ("t"), "Sample.GyroY"=w445, "Timeout"=0) -> (w452:T1)
          }
        }
      }
      frame "ReadSampleZ3" {
        n192 = xnode ("FIFO Method Node")("Timeout"=0) -> ("Element"=w456:u8, "Timed Out?"=w455:bool)  [unwired: 1 in, 1 out]
        n193 = case shown="False" w455 {
          tunnel: w456 -> [_ w465]
          tunnel: w454 -> [w459 w462]
          tunnel: [w458 w468] -> w453
          frame True {
            n194 = call "CheckGyroTimeout.vi"("GyroRxLoopData in"=w459) -> ("GyroRxLoopData out"=w458:T1)  [unwired: 10 in]
          }
          frame False {
            n195 = To Unsigned Long Integer(number=w465) -> (unsigned 32bit integer=w464:u32)
            n196 = xnode ("FIFO Method Node")("Element"=w465, "Timeout"=0) -> ()  [unwired: 1 in, 2 out]
            n197 = Logical Shift(y=i16 24, x=w464) -> (x << y=w461:u32)
            n198 = Bundle By Name(cluster=w462, "State"=GyroRxLoopStates."ReadSampleZ2" ("t"), "Sample.GyroZ"=w461, "Timeout"=0) -> (w468:T1)
          }
        }
      }
      frame "ReadSampleZ2" {
        n199 = xnode ("FIFO Method Node")("Timeout"=0) -> ("Element"=w472:u8, "Timed Out?"=w471:bool)  [unwired: 1 in, 1 out]
        n200 = case shown="False" w471 {
          tunnel: w472 -> [_ w483]
          tunnel: w470 -> [w475 w480]
          tunnel: [w474 w486] -> w469
          frame True {
            n201 = call "CheckGyroTimeout.vi"("GyroRxLoopData in"=w475) -> ("GyroRxLoopData out"=w474:T1)  [unwired: 10 in]
          }
          frame False {
            n202 = Unbundle By Name(w480) -> ("Sample.GyroZ"=w479:u32)
            n203 = To Unsigned Long Integer(number=w483) -> (unsigned 32bit integer=w482:u32)
            n204 = xnode ("FIFO Method Node")("Element"=w483, "Timeout"=0) -> ()  [unwired: 1 in, 2 out]
            n205 = Logical Shift(y=i16 16, x=w482) -> (x << y=w478:u32)
            n206 = Or(x=w479, y=w478) -> (x .or. y?=w477:u32)
            n207 = Bundle By Name(cluster=w480, "State"=GyroRxLoopStates."ReadSampleZ1" ("t"), "Sample.GyroZ"=w477, "Timeout"=0) -> (w486:T1)
          }
        }
      }
      frame "ReadSampleZ1" {
        n208 = xnode ("FIFO Method Node")("Timeout"=0) -> ("Element"=w490:u8, "Timed Out?"=w489:bool)  [unwired: 1 in, 1 out]
        n209 = case shown="False" w489 {
          tunnel: w490 -> [_ w501]
          tunnel: w488 -> [w493 w498]
          tunnel: [w492 w504] -> w487
          frame True {
            n210 = call "CheckGyroTimeout.vi"("GyroRxLoopData in"=w493) -> ("GyroRxLoopData out"=w492:T1)  [unwired: 10 in]
          }
          frame False {
            n211 = Unbundle By Name(w498) -> ("Sample.GyroZ"=w497:u32)
            n212 = To Unsigned Long Integer(number=w501) -> (unsigned 32bit integer=w500:u32)
            n213 = xnode ("FIFO Method Node")("Element"=w501, "Timeout"=0) -> ()  [unwired: 1 in, 2 out]
            n214 = Logical Shift(y=i16 8, x=w500) -> (x << y=w496:u32)
            n215 = Or(x=w497, y=w496) -> (x .or. y?=w495:u32)
            n216 = Bundle By Name(cluster=w498, "State"=GyroRxLoopStates."ReadSampleZ0" ("t"), "Sample.GyroZ"=w495, "Timeout"=0) -> (w504:T1)
          }
        }
      }
      frame "ReadSampleZ0" {
        n217 = xnode ("FIFO Method Node")("Timeout"=0) -> ("Element"=w508:u8, "Timed Out?"=w507:bool)  [unwired: 1 in, 1 out]
        n218 = case shown="False" w507 {
          tunnel: w508 -> [_ w518]
          tunnel: w506 -> [w511 w517]
          tunnel: [w510 w521] -> w505
          frame True {
            n219 = call "CheckGyroTimeout.vi"("GyroRxLoopData in"=w511) -> ("GyroRxLoopData out"=w510:T1)  [unwired: 10 in]
          }
          frame False {
            n220 = Unbundle By Name(w517) -> ("Sample.GyroZ"=w516:u32)
            n221 = To Unsigned Long Integer(number=w518) -> (unsigned 32bit integer=w515:u32)
            n222 = xnode ("FIFO Method Node")("Element"=w518, "Timeout"=0) -> ()  [unwired: 1 in, 2 out]
            n223 = Or(x=w516, y=w515) -> (x .or. y?=w514:u32)
            n224 = Bundle By Name(cluster=w517, "State"=GyroRxLoopStates."ReadSampleReserved" ("t"), "Sample.GyroZ"=w514, "ReservedCount"=u8 0, "Timeout"=0) -> (w521:T1)
          }
        }
      }
      frame "ReadSampleReserved" {
        n225 = xnode ("FIFO Method Node")("Timeout"=0) -> ("Element"=w526:u8, "Timed Out?"=w525:bool)  [unwired: 1 in, 1 out]
        n226 = case shown="False" w525 {
          tunnel: w526 -> [_ w539]
          tunnel: w524 -> [w529 w538]
          tunnel: [w528 w541] -> w523
          tunnel: w522 -> [_ w537]
          frame True {
            n227 = call "CheckGyroTimeout.vi"("GyroRxLoopData in"=w529) -> ("GyroRxLoopData out"=w528:T1)  [unwired: 10 in]
          }
          frame False {
            n228 = Increment(x=w537) -> (x+1=w536:u8)
            n229 = xnode ("FIFO Method Node")("Element"=w539, "Timeout"=0) -> ()  [unwired: 1 in, 2 out]
            n230 = Less?(x=w536, y=u8 12) -> (x < y?=w532:bool)
            n231 = Select(t=GyroRxLoopStates."ReadSampleReserved", s=w532, f=GyroRxLoopStates."ReadSampleStatus") -> (s? t:f=w533:T2)
            n232 = Bundle By Name(cluster=w538, "State"=w533, "ReservedCount"=w536, "Timeout"=0) -> (w541:T1)
          }
        }
      }
      frame "ReadSampleStatus" {
        n233 = xnode ("FIFO Method Node")("Timeout"=0) -> ("Element"=w545:u8, "Timed Out?"=w544:bool)  [unwired: 1 in, 1 out]
        n234 = case shown="False" w544 {
          tunnel: w545 -> [_ w550]
          tunnel: w543 -> [w548 w552]
          tunnel: [w547 w554] -> w542
          frame True {
            n235 = call "CheckGyroTimeout.vi"("GyroRxLoopData in"=w548) -> ("GyroRxLoopData out"=w547:T1)  [unwired: 10 in]
          }
          frame False {
            n236 = xnode ("FIFO Method Node")("Element"=w550, "Timeout"=0) -> ()  [unwired: 1 in, 2 out]
            n237 = Bundle By Name(cluster=w552, "State"=GyroRxLoopStates."ReadSampleSequenceNumber" ("t"), "Sample.Status"=w550, "Timeout"=0) -> (w554:T1)
          }
        }
      }
      frame "ReadSampleSequenceNumber" {
        n238 = xnode ("FIFO Method Node")("Timeout"=0) -> ("Element"=w558:u8, "Timed Out?"=w557:bool)  [unwired: 1 in, 1 out]
        n239 = case shown="False" w557 {
          tunnel: w558 -> [_ w563]
          tunnel: w556 -> [w561 w565]
          tunnel: [w560 w567] -> w555
          frame True {
            n240 = call "CheckGyroTimeout.vi"("GyroRxLoopData in"=w561) -> ("GyroRxLoopData out"=w560:T1)  [unwired: 10 in]
          }
          frame False {
            n241 = xnode ("FIFO Method Node")("Element"=w563, "Timeout"=0) -> ()  [unwired: 1 in, 2 out]
            n242 = Bundle By Name(cluster=w565, "State"=GyroRxLoopStates."ReadSampleTemperature1" ("t"), "Sample.SequenceNumber"=w563, "Timeout"=0) -> (w567:T1)
          }
        }
      }
      frame "ReadSampleTemperature1" {
        n243 = xnode ("FIFO Method Node")("Timeout"=0) -> ("Element"=w571:u8, "Timed Out?"=w570:bool)  [unwired: 1 in, 1 out]
        n244 = case shown="False" w570 {
          tunnel: w571 -> [_ w580]
          tunnel: w569 -> [w574 w577]
          tunnel: [w573 w583] -> w568
          frame True {
            n245 = call "CheckGyroTimeout.vi"("GyroRxLoopData in"=w574) -> ("GyroRxLoopData out"=w573:T1)  [unwired: 10 in]
          }
          frame False {
            n246 = To Word Integer(number=w580) -> (16bit integer=w579:i16)
            n247 = xnode ("FIFO Method Node")("Element"=w580, "Timeout"=0) -> ()  [unwired: 1 in, 2 out]
            n248 = Logical Shift(y=i16 8, x=w579) -> (x << y=w576:i16)
            n249 = Bundle By Name(cluster=w577, "State"=GyroRxLoopStates."ReadSampleTemperature0" ("t"), "Sample.Temperature"=w576, "Timeout"=0) -> (w583:T1)
          }
        }
      }
      frame "ReadSampleTemperature0" {
        n250 = xnode ("FIFO Method Node")("Timeout"=0) -> ("Element"=w587:u8, "Timed Out?"=w586:bool)  [unwired: 1 in, 1 out]
        n251 = case shown="False" w586 {
          tunnel: w587 -> [_ w596]
          tunnel: w585 -> [w590 w595]
          tunnel: [w589 w599] -> w584
          frame True {
            n252 = call "CheckGyroTimeout.vi"("GyroRxLoopData in"=w590) -> ("GyroRxLoopData out"=w589:T1)  [unwired: 10 in]
          }
          frame False {
            n253 = Unbundle By Name(w595) -> ("Sample.Temperature"=w594:i16)
            n254 = To Word Integer(number=w596) -> (16bit integer=w593:i16)
            n255 = xnode ("FIFO Method Node")("Element"=w596, "Timeout"=0) -> ()  [unwired: 1 in, 2 out]
            n256 = Or(x=w594, y=w593) -> (x .or. y?=w592:i16)
            n257 = Bundle By Name(cluster=w595, "State"=GyroRxLoopStates."ReadSampleCRC3" ("t"), "Sample.Temperature"=w592, "Timeout"=0) -> (w599:T1)
          }
        }
      }
      frame "ReadSampleCRC3" {
        n258 = xnode ("FIFO Method Node")("Timeout"=0) -> ("Element"=w603:u8, "Timed Out?"=w602:bool)  [unwired: 1 in, 1 out]
        n259 = case shown="False" w602 {
          tunnel: w603 -> [_ w614]
          tunnel: w601 -> [w606 w611]
          tunnel: [w605 w616] -> w600
          frame True {
            n260 = call "CheckGyroTimeout.vi"("GyroRxLoopData in"=w606) -> ("GyroRxLoopData out"=w605:T1)  [unwired: 10 in]
          }
          frame False {
            n261 = To Unsigned Long Integer(number=w614) -> (unsigned 32bit integer=w613:u32)
            n262 = xnode ("FIFO Method Node")("Element"=TRUE, "Timeout"=0) -> ()  [unwired: 1 in, 2 out]
            n263 = Logical Shift(y=i16 24, x=w613) -> (x << y=w610:u32)
            n264 = Bundle By Name(cluster=w611, "State"=GyroRxLoopStates."ReadSampleCRC2" ("t"), "CRC"=w610, "Timeout"=0) -> (w616:T1)
          }
        }
      }
      frame "ReadSampleCRC2" {
        n265 = xnode ("FIFO Method Node")("Timeout"=0) -> ("Element"=w621:u8, "Timed Out?"=w620:bool)  [unwired: 1 in, 1 out]
        n266 = case shown="False" w620 {
          tunnel: w621 -> [_ w632]
          tunnel: w619 -> [w624 w631]
          tunnel: [w623 w634] -> w618
          tunnel: w617 -> [_ w629]
          frame True {
            n267 = call "CheckGyroTimeout.vi"("GyroRxLoopData in"=w624) -> ("GyroRxLoopData out"=w623:T1)  [unwired: 10 in]
          }
          frame False {
            n268 = To Unsigned Long Integer(number=w632) -> (unsigned 32bit integer=w628:u32)
            n269 = Logical Shift(y=i16 16, x=w628) -> (x << y=w626:u32)
            n270 = Or(x=w629, y=w626) -> (x .or. y?=w630:u32)
            n271 = Bundle By Name(cluster=w631, "State"=GyroRxLoopStates."ReadSampleCRC1" ("t"), "CRC"=w630, "Timeout"=0) -> (w634:T1)
          }
        }
      }
      frame "ReadSampleCRC1" {
        n272 = xnode ("FIFO Method Node")("Timeout"=0) -> ("Element"=w639:u8, "Timed Out?"=w638:bool)  [unwired: 1 in, 1 out]
        n273 = case shown="False" w638 {
          tunnel: w639 -> [_ w650]
          tunnel: w637 -> [w642 w649]
          tunnel: [w641 w652] -> w636
          tunnel: w635 -> [_ w647]
          frame True {
            n274 = call "CheckGyroTimeout.vi"("GyroRxLoopData in"=w642) -> ("GyroRxLoopData out"=w641:T1)  [unwired: 10 in]
          }
          frame False {
            n275 = To Unsigned Long Integer(number=w650) -> (unsigned 32bit integer=w646:u32)
            n276 = Logical Shift(y=i16 8, x=w646) -> (x << y=w644:u32)
            n277 = Or(x=w647, y=w644) -> (x .or. y?=w648:u32)
            n278 = Bundle By Name(cluster=w649, "State"=GyroRxLoopStates."ReadSampleCRC0" ("t"), "CRC"=w648, "Timeout"=0) -> (w652:T1)
          }
        }
      }
      frame "ReadSampleCRC0" {
        n279 = xnode ("FIFO Method Node")("Timeout"=0) -> ("Element"=w657:u8, "Timed Out?"=w656:bool)  [unwired: 1 in, 1 out]
        n280 = case shown="False" w656 {
          tunnel: w657 -> [_ w666]
          tunnel: w655 -> [w660 w665]
          tunnel: [w659 w668] -> w654
          tunnel: w653 -> [_ w663]
          frame True {
            n281 = call "CheckGyroTimeout.vi"("GyroRxLoopData in"=w660) -> ("GyroRxLoopData out"=w659:T1)  [unwired: 10 in]
          }
          frame False {
            n282 = To Unsigned Long Integer(number=w666) -> (unsigned 32bit integer=w662:u32)
            n283 = Or(x=w663, y=w662) -> (x .or. y?=w664:u32)
            n284 = Bundle By Name(cluster=w665, "State"=GyroRxLoopStates."VerifyCRC" ("t"), "CRC"=w664, "Timeout"=0) -> (w668:T1)
          }
        }
      }
      frame "VerifyCRC" {
        n285 = xnode ("FIFO Method Node")("Timeout"=0) -> ("Element"=w673:u32, "Timed Out?"=w672:bool)  [unwired: 1 in, 1 out]
        n286 = case shown="False" w672 {
          tunnel: w673 -> [_ w680]
          tunnel: w671 -> [w675 w682]
          tunnel: [w675 w683] -> w670
          tunnel: w669 -> [_ w681]
          frame True {
          }
          frame False {
            n287 = Equal?(x=w681, y=w680) -> (x = y?=w676:bool)
            n288 = case shown="True" w676 {
              frame False {
              }
              frame True {
                n289 = xnode ("Register Read")() -> ("Data"=w685:u64)  [unwired: 1 in, 1 out]
                n290 = Increment(x=w685) -> (x+1=w684:u64)
                n291 = xnode ("Register Write")("Data"=w684) -> ()  [unwired: 1 in, 1 out]
              }
            }
            n292 = Select(t=GyroRxLoopStates."PrepareSample", s=w676, f=GyroRxLoopStates."ResponseCRCError" ("t")) -> (s? t:f=w677:T2)
            n293 = Bundle By Name(cluster=w682, "State"=w677) -> (w683:T1)
          }
        }
      }
      frame "PrepareSample" {
        n294 = xnode ("Register Read")() -> ("Data"=w689:u64)  [unwired: 1 in, 1 out]
        n295 = xnode ("Register Read")() -> ("Data"=w688:u64)  [unwired: 1 in, 1 out]
        n296 = xnode ("Register Read")() -> ("Data"=w687:u64)  [unwired: 1 in, 1 out]
        n297 = xnode ("Register Read")() -> ("Data"=w686:u64)  [unwired: 1 in, 1 out]
        n298 = Bundle By Name(cluster=w693, "State"=GyroRxLoopStates."MoveSample", "Sample.Timestamp"=w690, "Sample.TxBytes"=w689, "Sample.RxBytes"=w688, "Sample.TxFrames"=w687, "Sample.RxFrames"=w686) -> (w692:T1)
      }
      frame "MoveSample" {
        n299 = xnode ("FIFO Method Node")("Element"=w695, "Timeout"=0) -> ()  [unwired: 1 in, 2 out]
        n300 = Bundle By Name(cluster=w698, "State"=GyroRxLoopStates."ClearCRC") -> (w697:T1)
      }
      frame "ResponseHeaderError" {
        n301 = Bundle By Name(cluster=w702, "State"=GyroRxLoopStates."PrepareErrorCode", "ErrorSample.ErrorCode"=GyroErrorCodes."ResponseHeaderError" ("GyroErrorCodes")) -> (w701:T1)
      }
      frame "ResponseCRCError" {
        n302 = Bundle By Name(cluster=w706, "State"=GyroRxLoopStates."PrepareErrorCode", "ErrorSample.ErrorCode"=GyroErrorCodes."ResponseCRCError" ("GyroErrorCodes")) -> (w705:T1)
      }
      frame "ResponseTimeoutError" {
        n303 = Bundle By Name(cluster=w710, "State"=GyroRxLoopStates."PrepareErrorCode", "ErrorSample.ErrorCode"=GyroErrorCodes."ResponseTimeoutError" ("GyroErrorCodes")) -> (w709:T1)
      }
      frame "ResponseChecksumError" {
        n304 = Bundle By Name(cluster=w714, "State"=GyroRxLoopStates."PrepareErrorCode", "ErrorSample.ErrorCode"=GyroErrorCodes."ResponseChecksumError" ("GyroErrorCodes")) -> (w713:T1)
      }
      frame "PrepareErrorCode" {
        n305 = xnode ("Register Read")() -> ("Data"=w718:u64)  [unwired: 1 in, 1 out]
        n306 = xnode ("Register Read")() -> ("Data"=w717:u64)  [unwired: 1 in, 1 out]
        n307 = xnode ("Register Read")() -> ("Data"=w716:u64)  [unwired: 1 in, 1 out]
        n308 = xnode ("Register Read")() -> ("Data"=w715:u64)  [unwired: 1 in, 1 out]
        n309 = Bundle By Name(cluster=w722, "State"=GyroRxLoopStates."MoveErrorCode", "ErrorSample.Timestamp"=w719, "ErrorSample.TxBytes"=w718, "ErrorSample.RxBytes"=w717, "ErrorSample.TxFrames"=w716, "ErrorSample.RxFrames"=w715) -> (w721:T1)
      }
      frame "MoveErrorCode" {
        n310 = xnode ("FIFO Method Node")("Element"=w724, "Timeout"=0) -> ()  [unwired: 1 in, 2 out]
        n311 = Bundle By Name(cluster=w727, "State"=GyroRxLoopStates."ClearCRC") -> (w726:T1)
      }
      frame "ClearCRC" {
        n312 = xnode ("FIFO Method Node")("Element"=TRUE, "Timeout"=0) -> ()  [unwired: 1 in, 2 out]
        n313 = Bundle By Name(cluster=w732, "State"=GyroRxLoopStates."WaitForCRCCleared") -> (w731:T1)
      }
      frame "WaitForCRCCleared" {
        n314 = xnode ("FIFO Method Node")("Timeout"=0) -> ("Timed Out?"=w736:bool)  [unwired: 1 in, 2 out]
        n315 = Select(t=GyroRxLoopStates."WaitForCRCCleared", s=w736, f=GyroRxLoopStates."ReadHeader3" ("State")) -> (s? t:f=w733:T2)
        n316 = Bundle By Name(cluster=w739, "State"=w733) -> (w738:T1)
      }
    }
  }
  n317 = node-c288(w2) -> ()
